vi "PH_Sixpack.set periodic Interval.vi"(0 "VI in":refnum<vi>, 2 "PeriodicInterval [ms]":i32=10000, 5 "error in (no error)":errorcluster) -> (14 "VI out":refnum<vi>, 19 "error out":errorcluster)   [LabVIEW 2014, in "PH_Sixpack.lvlib"]
uses:
  PH_Sixpack.lvlib
  CS_Core/BaseProcess/BaseProcess.lvlib
  PH_Basics/PH_Common/PH_Common.lvlib
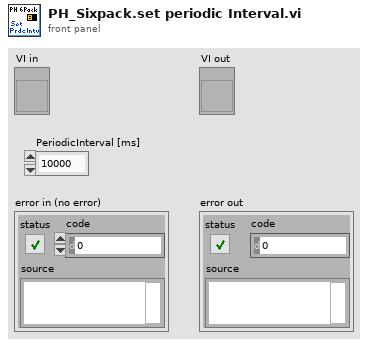
[diagram p1: front panel]
types:
  T1 = typedef "PH_Sixpack.lvlib/PH_Sixpack.i attribute.ctl" = cluster{"Information":cluster{"SixPack ID(0)":u16, "BaudRate(19200)":u16, "COM Port":enum32{"COM1", "COM2", "COM3", "COM4", "COM5", "COM6", "COM7", "COM8", "COM9"}, "HANDLE":i32}, "Serial Number":dbl, "Firmwareversion":dbl, "Axes":T2[], "Status":T14, "Axis to do a RefSearch":i32, "GUI Refs":cluster{"Information":refnum<vi>, "Serial Number":refnum<vi>, "Firmwareversion":refnum<vi>, "Status":refnum<vi>, "Axis to do a RefSearch":refnum<vi>, "Axes Configuration (Sixpack)":refnum<vi>, "Inputs":refnum<vi>, "PeriodicInterval [ms]":refnum<vi>}, "Constructor finished":bool, "Ignore Error":bool}
  T2 = typedef "PH_Sixpack.lvlib/PH_Sixpack.Axis Cluster.ctl" = cluster{"Config":T3, "To set?":cluster{"VmaxAmax":bool, "I max":bool, "VStartVminDivi":bool, "Ref Search Parameter":bool, "Stopswitch Limits":bool, "Axis Parameter":bool, "I Control":bool}}
  T3 = typedef "PH_Sixpack.lvlib/PH_Sixpack.Axis Configuration.ctl" = cluster{"VmaxAmax":T4, "I max (50%)":T5, "VStartVminDivi":T6, "Ref Search Parameter":T7, "Stopswitch Limits":T8, "Axis Parameter":T9, "I Control":T12}
  T4 = typedef "Sixpack - Driver.lvlib/VmaxAmax.ctl" = cluster{"VMax(511)":u16, "AMax(128)":u16}
  T5 = typedef "Sixpack - Driver.lvlib/PeakCurrent.ctl" = dbl
  T6 = typedef "Sixpack - Driver.lvlib/VStartVmin.ctl" = cluster{"VStart(5)":u16, "Vmin(4)":u16, "Div i (2)":enum8{"0", "1", "2", "3"}}
  T7 = typedef "Sixpack - Driver.lvlib/Ref Search Parameter.ctl" = cluster{"VRefMax(100)":u16, "DebouncingTime (22ms)":u8}
  T8 = typedef "Sixpack - Driver.lvlib/Stopswitch Limits.ctl" = cluster{"MinLeft(0)":u16, "MaxRight(1023)":u16}
  T9 = typedef "Sixpack - Driver.lvlib/Motor Parameter.ctl" = cluster{"Poslimit (6400)":u32, "P5 Bits":T10, "P6 Bits":T11}
  T10 = typedef "Sixpack - Driver.lvlib/MotorParameter_P5.ctl" = cluster{"MT_PI":bool, "MT_ROTARY":bool, "MT_AUTONULLCMD":bool, "MT_TESTNULL":bool, "MT_NULLLEFT":bool, "MT_NULLCENTRE":bool, "MT_STOPNULL":bool, "MT_FILTERSWITCH":bool}
  T11 = typedef "Sixpack - Driver.lvlib/MotorParameter_P6.ctl" = cluster{"MT_OPTIMIZEWAY":bool, "MT_FASTREF":bool, "MT_MECHREF":bool, "MT_DELAYTESTNULL":bool, "MT_STOPSOFT":bool, "MT_STOPNOREF":bool, "MT_NULLPOSITIVE":bool, "MUT_STOPFULSTEPS":bool}
  T12 = typedef "Sixpack - Driver.lvlib/Current Control.ctl" = cluster{"PowerDownDelay (500)":u16, "PowerDown (0%)":T13, "Standing (50%)":T13, "Running (75%)":T13, "Accelerating (100%)":T13}
  T13 = typedef "Sixpack - Driver.lvlib/Current.ctl" = enum8{"100%", "75%", "50%", "38%", "25%", "19%", "13%", "9%", "0%"}
  T14 = typedef "PH_Sixpack.lvlib/PH_Sixpack.Status.ctl" = enum32{"None", "Init", "Configure", "configured", "Close", "closed"}
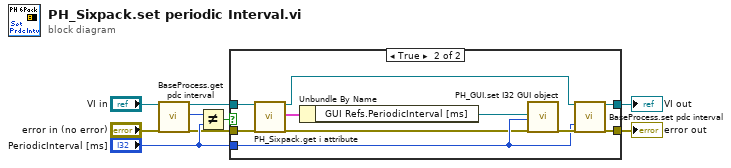
[diagram p0: block diagram]
diagram:
  n1 = call "BaseProcess.get pdc interval.vi"("i ref in"="VI in", "error in (no error)"="error in (no error)") -> ("i ref out"=w6:refnum<vi>, "PeriodicInterval"=w7:i32, "error out"=w4:errorcluster)  [unwired: 15 in]
  n2 = Not Equal?(x=w7, y="PeriodicInterval [ms]") -> (x != y?=w9:bool)
  n3 = case shown="True" w9 {
    tunnel: [w10 w21] -> w2
    tunnel: [w11 w20] -> w3
    tunnel: w4 -> [w10 w15]
    tunnel: w6 -> [w11 w17]
    tunnel: "PeriodicInterval [ms]" -> [_ w18]
    frame False {
    }
    frame True {
      n4 = call "PH_Sixpack.get i attribute.vi"("i ref in"=w17, "error in (no error)"=w15) -> ("i ref out"=w16:refnum<vi>, "i attribute"=w13:T1, "error out"=w14:errorcluster)  [unwired: 15 in]
      n5 = Unbundle By Name(w13) -> ("GUI Refs.PeriodicInterval [ms]"=w12:refnum<vi>)
      n6 = call "PH_GUI.set I32 GUI object.vi"("I32 GUI Ref"=w12, "value"=w18, "error in (no error)"=w14) -> ("error out"=w19:errorcluster)  [unwired: 16 in]
      n7 = call "BaseProcess.set pdc interval.vi"("i ref in"=w16, "PeriodicInterval [ms]"=w18, "error in (no error)"=w19) -> ("i ref out"=w20:refnum<vi>, "error out"=w21:errorcluster)  [unwired: 14 in, 1 out]
    }
  }
  "VI out" <- w3
  "error out" <- w2
